vi "reqstTask_quit.vi"(8 "error in (no error)":errorcluster, 11 "TaskRef in":refnum<vi>) -> (0 "error IO":errorcluster, 3 "TaskRef out":refnum<vi>)   [LabVIEW 2015, in "pdbm_task_route.lvlib"]
uses:
  pdbm_task_route.lvlib
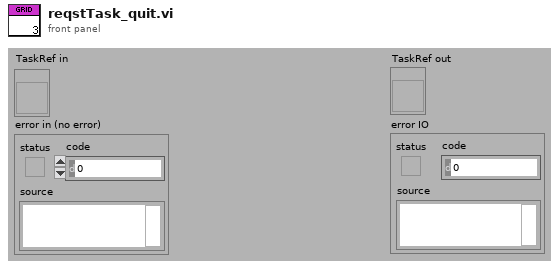
[diagram p1: front panel]
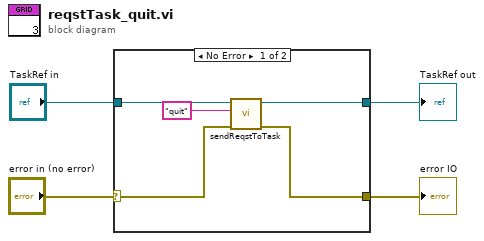
[diagram p0: block diagram]
diagram:
  n1 = case shown="No Error" "error in (no error)" {
    selector: "error in (no error)" -> [w6 w10]
    tunnel: "TaskRef in" -> [w9 w11]
    tunnel: [w8 w11] -> w3
    tunnel: [w5 w10] -> w1
    frame No Error {
      n2 = call "sendReqstToTask.vi"("error in (no error)"=w6, "request"="quit", "TaskRef in"=w9) -> ("error IO"=w5:errorcluster, "TaskRef out"=w8:refnum<vi>)  [unwired: 7 in]
    }
    frame Error {
    }
  }
  "TaskRef out" <- w3
  "error IO" <- w1
